vi "SPI API - R-Series FGPA Main.vi"() -> ()   [LabVIEW 2015]
doc: "This is the main FPGA VI for the SPI application. It sets up the SPI communication and then runs the SPI engine. In a parallel loop, data is continually read from the Real Time application and sent to the SPI engine. The SPI engine handles all communication between the FPGA and the SPI chip."
uses:
  <userlib>/_NI SPI IP/FPGA/Controllers/Public/Transfer Settings.ctl
  <vilib>/Platform/TimedLoop/XDataNode/timing_clust.ctl
  <vilib>/Platform/TimedLoop/XDataNode/nitl_modes.ctl
  <vilib>/Platform/TimedLoop/XDataNode/wakeup.ctl
  vi.lib/SPIAPI/Controls/SPI API DIO Lines.ctl
  <vilib>/rvi/Emulation/niFpgaGetClockAttributes.vi
  <vilib>/rvi/Emulation/niFpgaSctlEmulationGetInTimedLoop.vi
  <vilib>/rvi/Emulation/niFpgaEmulationReportErrorSimple.vi
  <vilib>/rvi/Emulation/niFpgaCriticalErrorInLSC.vi
  <vilib>/Platform/TimedLoop/XDataNode/XDataNode.xnode
  <vilib>/Platform/TimedLoop/XDataNode/XDNodeRunTimeDep.lvlib
  <userlib>/_NI SPI IP/FPGA/Controllers/NI SPI IP FPGA.lvlib
panel:
  out "Response from Slave":u64
  out "read Iterations":i32
  in  "Data To Slave":u64=2147483648
  in  "Chip Select":u8
  in  "SPI PHY Settings":T1={"Divide Value"=20, "Transfer Length (bits)"=32, "CS Asserted Polarity"=FALSE, "Clock Polarity (CPOL)"=FALSE, "Clock Phase (CPHA)"=FALSE, "Lengthen MISO Setup"=FALSE, "Direction Change Bit"=0, "MOSI Starts as Output"=FALSE, "Tristatable MOSI"=FALSE} {"Direction Change Bit" max=64 step=1; "Transfer Length (bits)" min=1 max=64 step=1}
  in  "Data Rate (S/s)":u32=10000
  out "oclk freq":u32
  out "oclk div":u32
  out "FPGA Error":errorcluster
  out "Actual Loop Ticks":u32
  # "Overview: This is the FPGA VI that communicates with the MAX5216.\nRequirements: LabVIEW Full Development System, LabVIEW Real Time,  LabVIEW FPGA, MAX5216, NI System on Module, NI 9651.\nInstructions:\nRun RT Main without making adjustments to this VI to avoid a recompile.  If you desire to adjust this VI, do so, \nthen be sure to point RT Main to this VI instead of the pre-compiled bitfile that it currently targets."
  # "OUTPUT"
  # "INPUT"
  # "ADC Data::Debug"
  # "Acquisition Parameters"
  # "SPI PHY Settings"
  # "Debug"
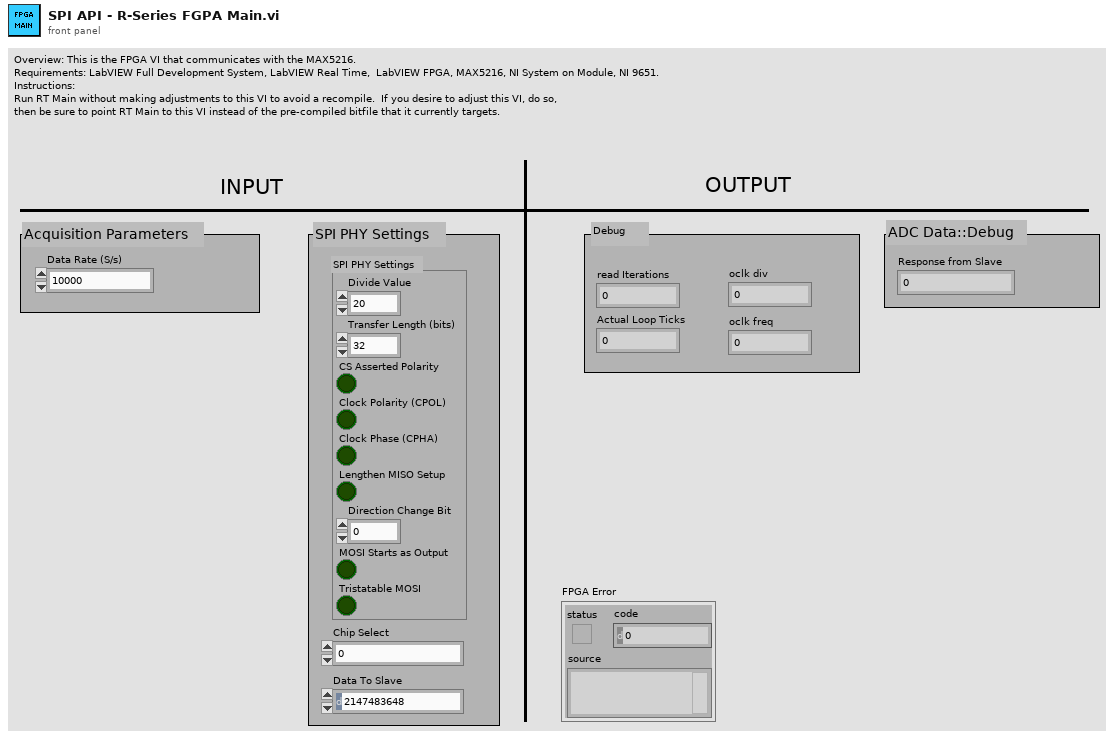
[diagram p1: front panel]
types:
  T1 = typedef "NI SPI IP FPGA.lvlib/Transfer Settings.ctl" = cluster{"Divide Value":u8, "Transfer Length (bits)":u8, "CS Asserted Polarity":bool, "Clock Polarity (CPOL)":bool, "Clock Phase (CPHA)":bool, "Lengthen MISO Setup":bool, "Direction Change Bit":u8, "MOSI Starts as Output":bool, "Tristatable MOSI":bool}
  T2 = typedef "SPI API DIO Lines.ctl" = cluster{"SCLK":refnum<k21>, "MISO":refnum<k21>, "MOSI":refnum<k21>, "CS 0":refnum<k21>, "CS 1":refnum<k21>, "CS 2":refnum<k21>, "CS 3":refnum<k21>, "CS 4":refnum<k21>, "CS 5":refnum<k21>}
  T3 = typedef "SPI Digital IO Lines.ctl" = cluster{"SCLK":refnum<k21>, "MISO":refnum<k21>, "MOSI":refnum<k21>, "CS 0":refnum<k21>, "CS 1":refnum<k21>, "CS 2":refnum<k21>, "CS 3":refnum<k21>, "CS 4":refnum<k21>, "CS 5":refnum<k21>}
  T4 = typedef "SPI API References.ctl" = cluster{"DLU To SPI Engine Data FIFO":refnum<k21>, "SPI Engine to DLU Data FIFO":refnum<k21>, "Data to SPI Engine (Cache) Register":refnum<k21>, "SPI Settings to SPI Engine (Cache) Register":refnum<k21>}
  T5 = typedef "XDNodeRunTimeDep.lvlib/timing_clust.ctl" = cluster{"Expected End [f-1]":u64, "Actual End [f-1]":u64, "Finished Late? [f-1]":bool, "Expected End [i-1]":u64, "Actual End [i-1]":u64, "Finished Late? [i-1]":bool, "Expected Start [i]":u64, "Actual Start [i]":u64, "Expected Start [f]":u64, "Actual Start [f]":u64, "Source Name":string, "Structure Name":string, "Period":i64, "Deadline":i64, "Offset":i64, "Start":i64, "Priority":i32, "Timeout":i32, "Mode":T6, "Wakeup Reason":T7, "Error":errorcluster, "Source Type":string, "Secondary Source Type":string, "Global End Time":u64, "Global Start Time":u64, "Frame Duration":u64, "Iteration Duration":u64, "Assigned CPU":i32, "I/O Scan Engine Mode":u32}
  T6 = typedef "XDNodeRunTimeDep.lvlib/nitl_modes.ctl" = enum32{"No Change", "Process missed periods, maintain original phase", "Discard missed periods, maintain original phase", "Process missed periods, ignore original phase", "Discard missed periods, ignore original phase"}
  T7 = typedef "XDNodeRunTimeDep.lvlib/wakeup.ctl" = enum32{"Normal", "Aborted", "Asynchronous wakeup", "Timing source error", "Timed loop error", "Timeout"}
  T8 = typedef "SPI API Response Data.ctl" = cluster{"Data to Node":u64, "Node Id":u16}
  T9 = typedef "NI SPI IP FPGA.lvlib/Spi Master Inputs.ctl" = cluster{"MISO":bool}
  T10 = typedef "NI SPI IP FPGA.lvlib/Spi Master Outputs.ctl" = cluster{"Chip Select":bool, "Clock":bool, "MOSI":bool, "MOSI OE":bool}
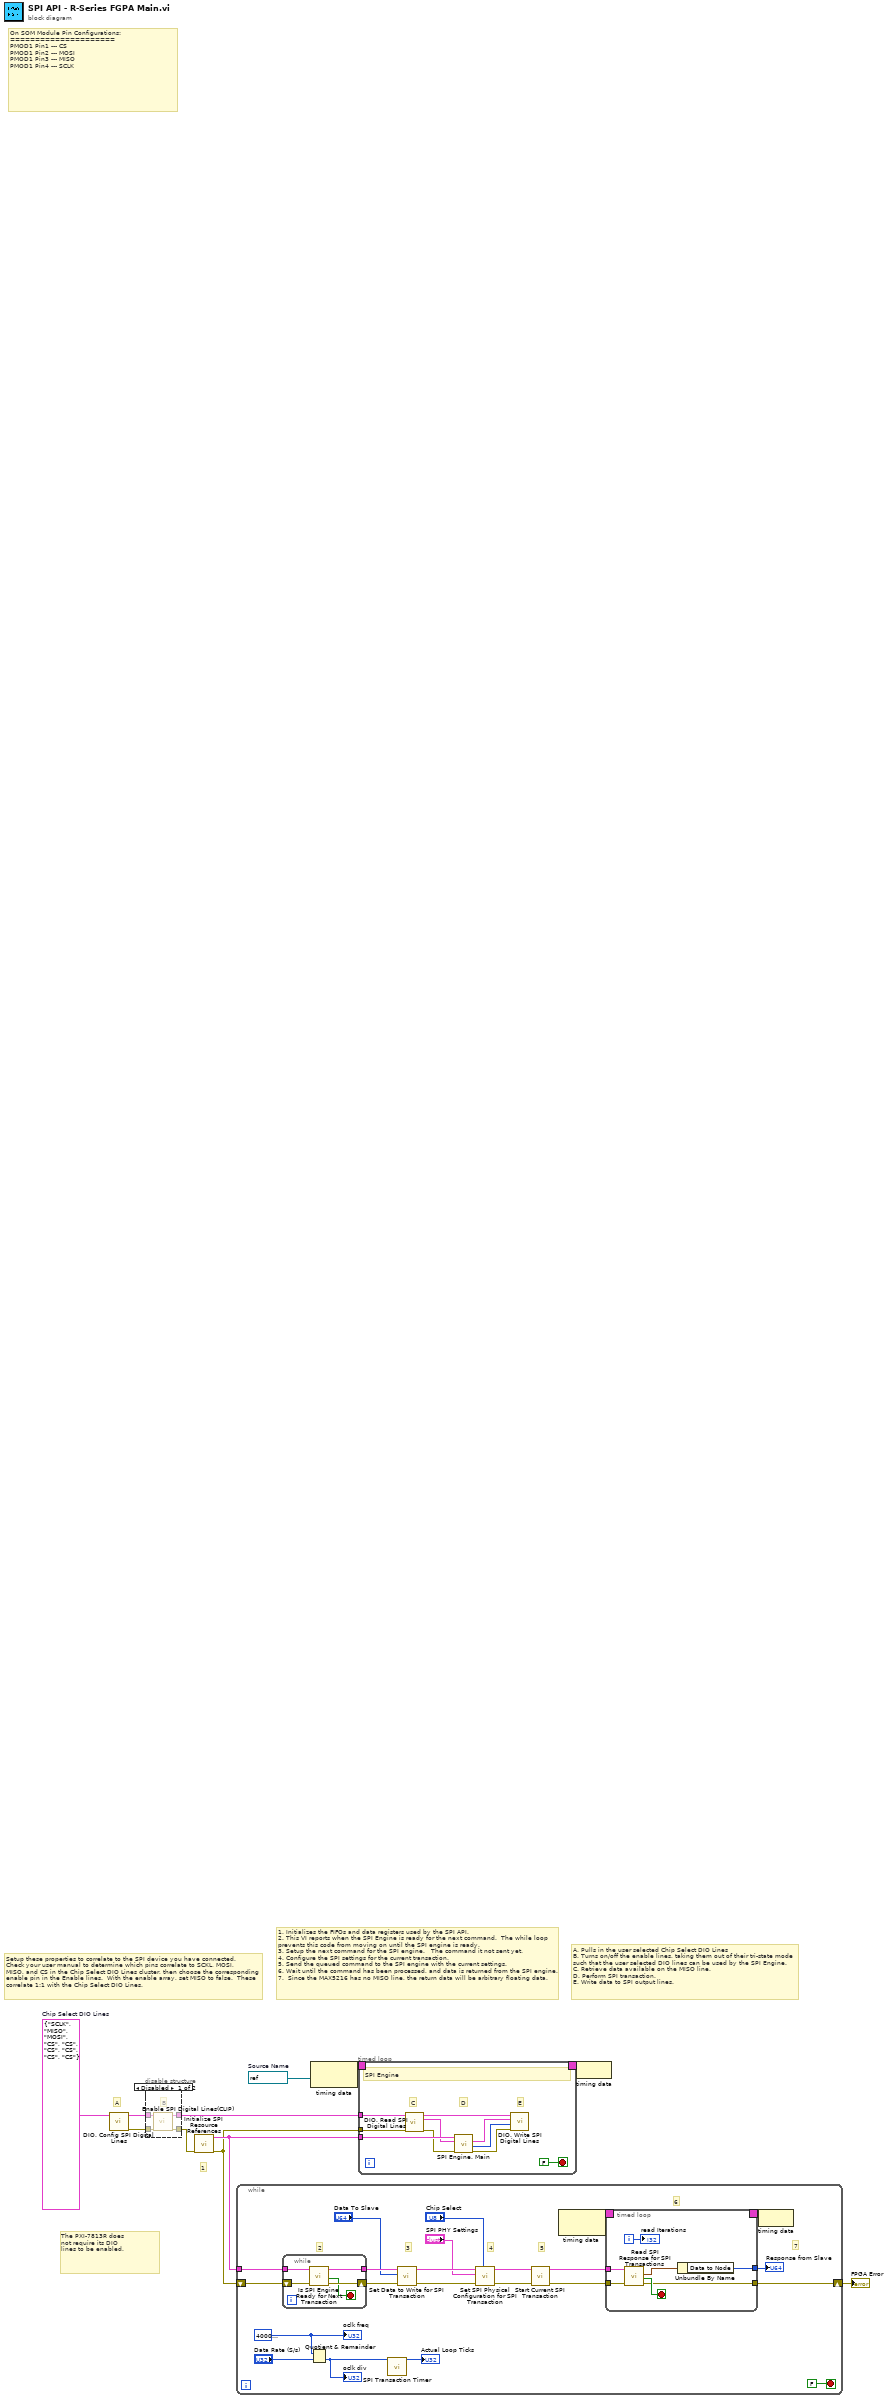
[diagram p0: block diagram]
diagram:
  w7 = T2 {"SCLK"="SCLK", "MISO"="MISO", "MOSI"="MOSI", "CS 0"="CS", "CS 1"="CS", "CS 2"="CS", "CS 3"="CS", "CS 4"="CS", "CS 5"="CS"}  # Chip Select DIO Lines
  w8 = refnum<k21> "80MHz"  # Source Name
  # "The PXI-7813R does\nnot require its DIO \nlines to be enabled."
  # "A. Pulls in the user selected Chip Select DIO Lines\nB. Turns on/off the enable lines, taking them out of their tri-state mode \nsuch that the user selected DIO lines can be used by the SPI Engine.\nC. Retrieve data available on the MISO line.\nD. Perform SPI transaction.\nE. Write data to SPI output lines."
  # "A"
  # "1. Initializes the FIFOs and data registers used by the SPI API.\n2. This VI reports when the SPI Engine is ready for the next command.  The while loop \nprevents this code from moving on until the SPI engine is ready.\n3. Setup the next command for the SPI engine.   The command it not sent yet.\n4. Configure the SPI settings for the current transaction.\n5. Send the queued command to the SPI engine with the current settings.\n6. Wait until the command has been processed, and data is returned from the SPI engine.\n7.  Since the MAX5216 has no MISO line, the return data will be arbitrary floating data."
  # "1"
  # "Setup these properties to correlate to the SPI device you have connected.\nCheck your user manual to determine which pins correlate to SCKL, MOSI,\nMISO, and CS in the Chip Select DIO Lines cluster, then choose the corresponding\nenable pin in the Enable lines.  With the enable array, set MISO to false.  These\ncorrelate 1:1 with the Chip Select DIO Lines."
  # "On SOM Module Pin Configurations:\n=====================\nPMOD1 Pin1 --- CS\nPMOD1 Pin2 --- MOSI\nPMOD1 Pin3 --- MISO\nPMOD1 Pin4 --- SCLK"
  n1 = call "DIO. Config SPI Digital Lines.vi"("SPI DIO Lines"=w7) -> ("error out"=w3:errorcluster, "Chip Select DIO Lines"=w4:T2)  [unwired: 9 in]
  n2 = disable-structure shown="Disabled" {
    disable-tunnel: w4 -> [w15 w17]
    disable-tunnel: w3 -> [w14 w16]
    disable-tunnel: [w13 w17] -> w2
    disable-tunnel: [w12 w16] -> w1
    frame Disabled {
      # "B"
      n3 = call <vilib>:"Enable SPI Digital Lines(CLIP).vi"("error in"=w14, "SPI DIO Lines"=w15) -> ("error out"=w12:errorcluster, "Chip Select DIO Lines"=w13:T3)  [unwired: 8 in]
    }
    frame Enabled {
    }
  }
  n4 = call "Initialize SPI Resource References.vi"("error in"=w1) -> ("error out"=w5:errorcluster, "SPI API References"=w9:T4)  [unwired: 9 in]
  n5 = while {
    shift-right: [w24] -> w6
    shift-left: w5 -> [w35]
    tunnel: w9 -> [w36]
    stop <- FALSE stop-if-true
    w20 = u32 40000000 ("oclk freq")
    # "7"
    # "6"
    # "5"
    # "4"
    # "3"
    # "2"
    n6 = while {
      shift-right: [w44] -> w38
      shift-left: w35 -> [w41]
      tunnel: w36 -> [w42]
      tunnel: [w43] -> w37
      stop <- w40 stop-if-true
      n7 = call "Is SPI Engine Ready for Next Transaction.vi"("error in"=w41, "Private Data In"=w42) -> ("error out"=w44:errorcluster, "SPI Channel Ready"=w40:bool, "Private Data Out"=w43:T4)  [unwired: 6 in, 1 out]
    }
    n8 = Quotient & Remainder(x=w20, y="Data Rate (S/s)") -> (floor(x/y)=w18:u32)  [unwired: 1 out]
    "oclk div" <- w18
    n9 = call "SPI Transaction Timer.vi"("Loop Time (Ticks)"=w18) -> ("Actual Time (Ticks)"=→"Actual Loop Ticks":u32)  [unwired: 10 in]
    n10 = call "Set Data to Write for SPI Transaction.vi"("error in"=w38, "Data In"="Data To Slave", "Private Data In"=w37) -> ("error out"=w30:errorcluster, "Private Data Out"=w31:T4)  [unwired: 7 in]
    n11 = call "Set SPI Physical Configuration for SPI Transaction.vi"("Chip Select"="Chip Select", "error in"=w30, "SPI Physical Settings"="SPI PHY Settings", "Private Data In"=w31) -> ("error out"=w27:errorcluster, "Private Data Out"=w28:T4)  [unwired: 6 in]
    n12 = call "Start Current SPI Transaction.vi"("error in"=w27, "Private Data In"=w28) -> ("error out"=w32:errorcluster, "Private Data Out"=w26:T4)  [unwired: 7 in, 1 out]
    n13 = node-c288() -> (w34:T5)  [unwired: 1 in]
    n14 = timed-loop {
      timing: w34 -> [_]
      timing-out: [_] -> w33
      tunnel: w32 -> [w51]
      tunnel: w26 -> [w50]
      tunnel: [w45] -> w23
      tunnel: [w47] -> w24
      i -> [w46]
      stop <- w49 stop-if-true
      n15 = call "Read SPI Response for SPI Transactions.vi"("error in"=w51, "Private Data In"=w50) -> ("error out"=w47:errorcluster, "Read Data Valid?"=w49:bool, "Read Data"=w48:T8)  [unwired: 6 in, 1 out]
      n16 = Unbundle By Name(w48) -> ("Data to Node"=w45:u64)
      "read Iterations" <- w46
    }
    "Response from Slave" <- w23
    n17 = node-c288(w33) -> ()
    "oclk freq" <- w20
  }
  "FPGA Error" <- w6
  n18 = node-c288(w8) -> (w11:T5)
  n19 = timed-loop {
    tunnel: w9 -> [w63]
    tunnel: w5 -> [w61]
    tunnel: w2 -> [w64]
    timing: w11 -> [_]
    timing-out: [_] -> w10
    stop <- FALSE stop-if-true
    # "E"
    # "D"
    # "C"
    # "SPI Engine"
    n20 = call "DIO. Read SPI Digital Lines.vi"("Chip Select DIO Lines"=w64, "error in"=w61) -> ("Chip Select DIO Lines Out"=w65:T2, "SPI Read Data"=w62:T9, "error out"=w56:errorcluster)  [unwired: 11 in]
    n21 = call "SPI Engine. Main.vi"("error in"=w56, "SPI Read Data"=w62, "SPI API References"=w63) -> ("error out"=w58:errorcluster, "Chip Select ID"=w57:u8, "SPI DIO Output"=w60:T10)  [unwired: 5 in, 1 out]
    n22 = call "DIO. Write SPI Digital Lines.vi"("error in"=w58, "CS Index"=w57, "spi output"=w60, "Chip Select DIO Lines"=w65) -> ()  [unwired: 6 in, 2 out]
  }
  n23 = node-c288(w10) -> ()
